vi "Sift for Intrinsic Mode Function.vi"(5 "Max Iterations (1000)":i32=1000, 7 "Tolerance (1e-9)":dbl=1e-09 format="%#_13g", 11 "Waveform":waveform(dbl)) -> (3 "IMF":waveform(dbl))   [LabVIEW 2013, in "Empirical Mode Decomposition.lvlib"]
uses:
  Empirical Mode Decomposition.lvlib
panel:
  out "Std Dev":dbl
  out "Sifting Iterations":i32
  out "h1k":waveform(dbl)(graph)
  out "m1k":waveform(dbl)(graph)
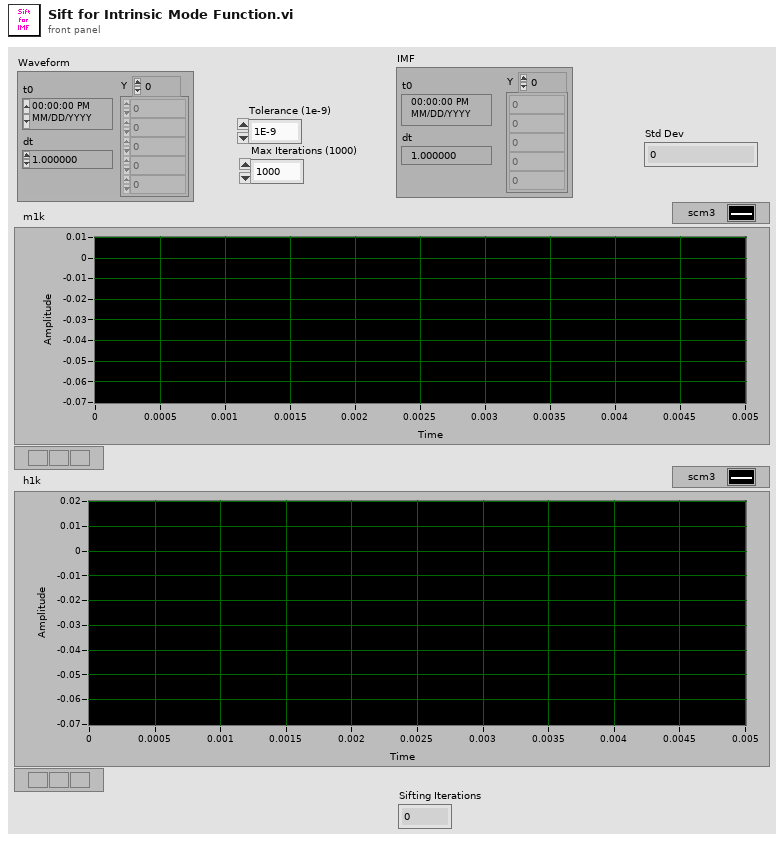
[diagram p1: front panel]
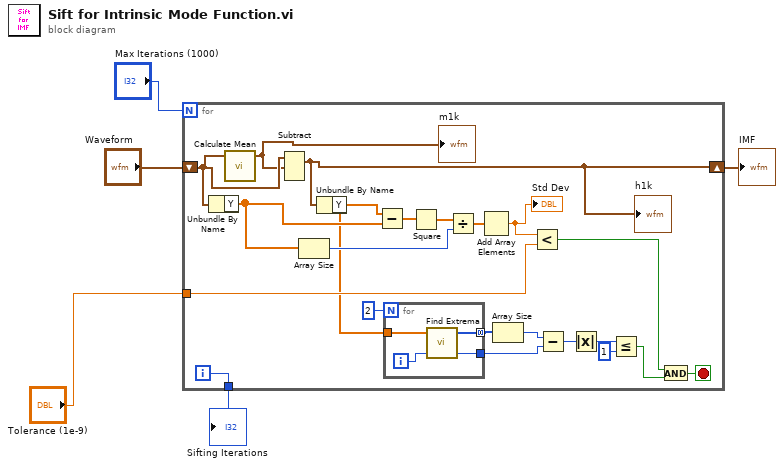
[diagram p0: block diagram]
diagram:
  n1 = for {
    N: "Max Iterations (1000)" -> [_]
    shift-right: [w19] -> w4
    shift-left: "Waveform" -> [w18]
    tunnel: [w27] -> w2
    tunnel: "Tolerance (1e-9)" -> [w22]
    i -> [w27]
    stop <- w14 stop-if-true
    n2 = Unbundle By Name(w18) -> ("Y"=w21:dbl[])
    n3 = call "Calculate Mean.vi"("Waveform"=w18) -> ("Waveform Mean"=w11:waveform(dbl))  [unwired: 4 in]
    "m1k" <- w11
    n4 = Subtract(1:w11, 2:w18) -> (0:w19:waveform(dbl))  [unwired: 1 in, 1 out]
    "h1k" <- w19
    n5 = Array Size(array=w21) -> (size(s)=w20:i32)
    n6 = Unbundle By Name(w19) -> ("Y"=w6:dbl[])
    n7 = Subtract(x=w6, y=w21) -> (x-y=w26:dbl[])
    n8 = for {
      N: 2 -> [_]
      tunnel: w6 -> [w30]
      tunnel: [w29] -> w8
      tunnel: [w28] -> w10 mode=concatenating
      i -> [w31]
      n9 = call "Find Extrema.vi"("peaks/valleys"=w31, "Array"=w30) -> ("# Zero Crossings"=w29:i32, "Indicies"=w28:u32[])  [unwired: 1 in, 1 out]
    }
    n10 = Square(x=w26) -> (x^2=w25:dbl[])
    n11 = Divide(x=w25, y=w20) -> (x/y=w24:dbl[])
    n12 = Add Array Elements(numeric array=w24) -> (sum=w23:dbl)
    "Std Dev" <- w23
    n13 = Array Size(array=w10) -> (size(s)=w9:i32)
    n14 = Less?(x=w23, y=w22) -> (x < y?=w12:bool)
    n15 = Subtract(x=w9, y=w8) -> (x-y=w17:i32)
    n16 = Absolute Value(x=w17) -> (abs(x)=w16:i32)
    n17 = Less Or Equal?(x=w16, y=1) -> (x <= y?=w13:bool)
    n18 = And(x=w12, y=w13) -> (x .and. y?=w14:bool)
  }
  "Sifting Iterations" <- w2
  "IMF" <- w4
